vi "Dymin_FPGA_Main.vi"() -> ()   [LabVIEW 2016]
doc: "This VI demonstrates how to use an external signal to control the execution rate of a while loop."
uses:
  <vilib>/Platform/TimedLoop/XDataNode/timing_clust.ctl
  <vilib>/Platform/TimedLoop/XDataNode/nitl_modes.ctl
  <vilib>/Platform/TimedLoop/XDataNode/wakeup.ctl
  <vilib>/rvi/Emulation/niFpgaGetClockAttributes.vi
  <vilib>/rvi/Emulation/niFpgaSctlEmulationGetInTimedLoop.vi
  <vilib>/rvi/Emulation/niFpgaEmulationReportErrorSimple.vi
  <vilib>/rvi/eio/common/nirviEmuTemplateMethod_errors.vi
  <vilib>/rvi/Emulation/niFpgaCriticalErrorInLSC.vi
  <vilib>/rvi/Emulation/niFpgaEmulationIsFPGAContextNoSignature.vi
  <vilib>/rvi/errors/niFpgaSetErrorForExecOnDevCompSimple.vi
  <vilib>/rvi/eio/common/nirviEmuReportErrorAndStop.vi
  <vilib>/rvi/DataTransferAndStorage/Container/Common/niFpgaContainerGetUniqueNameForEmu.vi
  <vilib>/rvi/FIFO/Fifo_Resource/nirvififoEmulationSetSize.vi
  <vilib>/rvi/FIFO/Fifo_Resource/nirviFifoEmulationQueueMgr.vi
  <instcachedir>/0/nirviFifoEmulationQueueMgr_E5CAEC123FF24DC58D834DCA3CDAA9B5.lvgen/nirviFifoEmulationQueueMgr_E5CAEC123FF24DC58D834DCA3CDAA9B5_001.vi
  <vilib>/rvi/FIFO/Fifo_Resource/nirvififoEmulationDetermineInputValidOut.vi
  <vilib>/rvi/FIFO/Fifo_Resource/nirvififoEmulationCreateLock.vi
  <vilib>/rvi/Emulation/niFpgaProcessEmulError.vi
  <vilib>/rvi/FIFO/Fifo_Resource/nirvififoEmulationObtainLock.vi
  <vilib>/rvi/FIFO/Fifo_Resource/nirvififoEmulationReleaseLock.vi
  <vilib>/rvi/occurrence/nirviWaitOnOccurrenceBase.vi
  <vilib>/rvi/errors/nirviReportUnexpectedCaseInternalError.vi
  <vilib>/rvi/errors/nirviReportUnexpectedCaseInternalError (U32).vi
  <vilib>/Utility/error.llb/Clear Errors.vi
  <vilib>/rvi/interface/RandomDataEmulation/niFpgaRandomDataHandleErrors.vi
  <vilib>/eio/EIONode/EIONode.xnode
  <vilib>/Platform/TimedLoop/XDataNode/XDataNode.xnode
  <vilib>/rvi/DataTransferAndStorage/Container/XNode/niFpgaContainer.xnode
  <vilib>/rvi/FIFO/Fifo_Resource/nirvififoEmulationWrite.vi
  <vilib>/rvi/FIFO/Fifo_Resource/nirvififoEmulationRead.vi
  <vilib>/rvi/interface/RandomDataEmulation/nirviRandomDataFpgaReadWriteTemplate.vi
  <vilib>/Platform/TimedLoop/XDataNode/XDNodeRunTimeDep.lvlib
panel:
  in  "T3":u32=1000
  in  "T2":u32=1000
  in  "T1":u32=1000
  in  "T0":u32=1000
  in  "t3":u32=1000
  in  "t2":u32=1000
  in  "t1":u32=1000
  in  "t0":u32=1000
  in  "V3":u16=1000
  in  "V2":i16=1000
  in  "V1":i16=232
  in  "V0":u16=1000
  out "Overflow1":bool
  in  "Upper Threhold (counts)":u32
  out "Overflow2":bool
  out "PIX CLK (bits)":u32
  in  "Dymin On?":bool
  in  "stop 4":bool
  in  "stop 3":bool
  in  "stop 2":bool
  in  "stop 1":bool
  # "Reminder:These \"Volts\" are actually in bits.  Use  the RT_Main vi to run this code by inputting actual Volts.  Floats aren't possible in an FPGA program."
  # "Step before step with tn=0 is the last Dymin Step, threshold is ignored on last step, just count APD counts in selected time"
  # "AOM Voltage (bits)"
  # "Times (#80MHz periods)"
  # "Threshold (counts)"
  # "16=200ns\n32=400ns"
  # "nominal 12 bit ADC volts"
  # ".1=82\n.2=164\n.3=246"
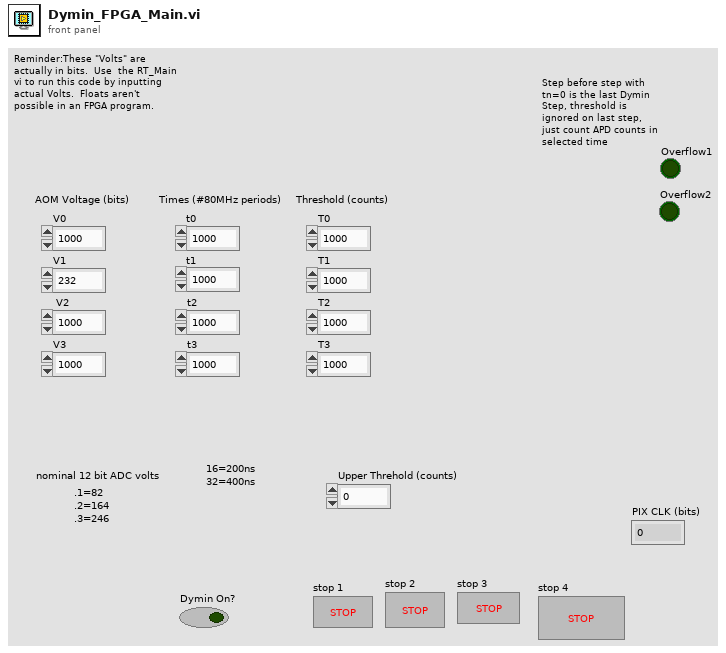
[diagram p1: front panel]
types:
  T1 = typedef "XDNodeRunTimeDep.lvlib/timing_clust.ctl" = cluster{"Expected End [f-1]":u64, "Actual End [f-1]":u64, "Finished Late? [f-1]":bool, "Expected End [i-1]":u64, "Actual End [i-1]":u64, "Finished Late? [i-1]":bool, "Expected Start [i]":u64, "Actual Start [i]":u64, "Expected Start [f]":u64, "Actual Start [f]":u64, "Source Name":string, "Structure Name":string, "Period":i64, "Deadline":i64, "Offset":i64, "Start":i64, "Priority":i32, "Timeout":i32, "Mode":T2, "Wakeup Reason":T3, "Error":errorcluster, "Source Type":string, "Secondary Source Type":string, "Global End Time":u64, "Global Start Time":u64, "Frame Duration":u64, "Iteration Duration":u64, "Assigned CPU":i32, "I/O Scan Engine Mode":u32}
  T2 = typedef "XDNodeRunTimeDep.lvlib/nitl_modes.ctl" = enum32{"No Change", "Process missed periods, maintain original phase", "Discard missed periods, maintain original phase", "Process missed periods, ignore original phase", "Discard missed periods, ignore original phase"}
  T3 = typedef "XDNodeRunTimeDep.lvlib/wakeup.ctl" = enum32{"Normal", "Aborted", "Asynchronous wakeup", "Timing source error", "Timed loop error", "Timeout"}
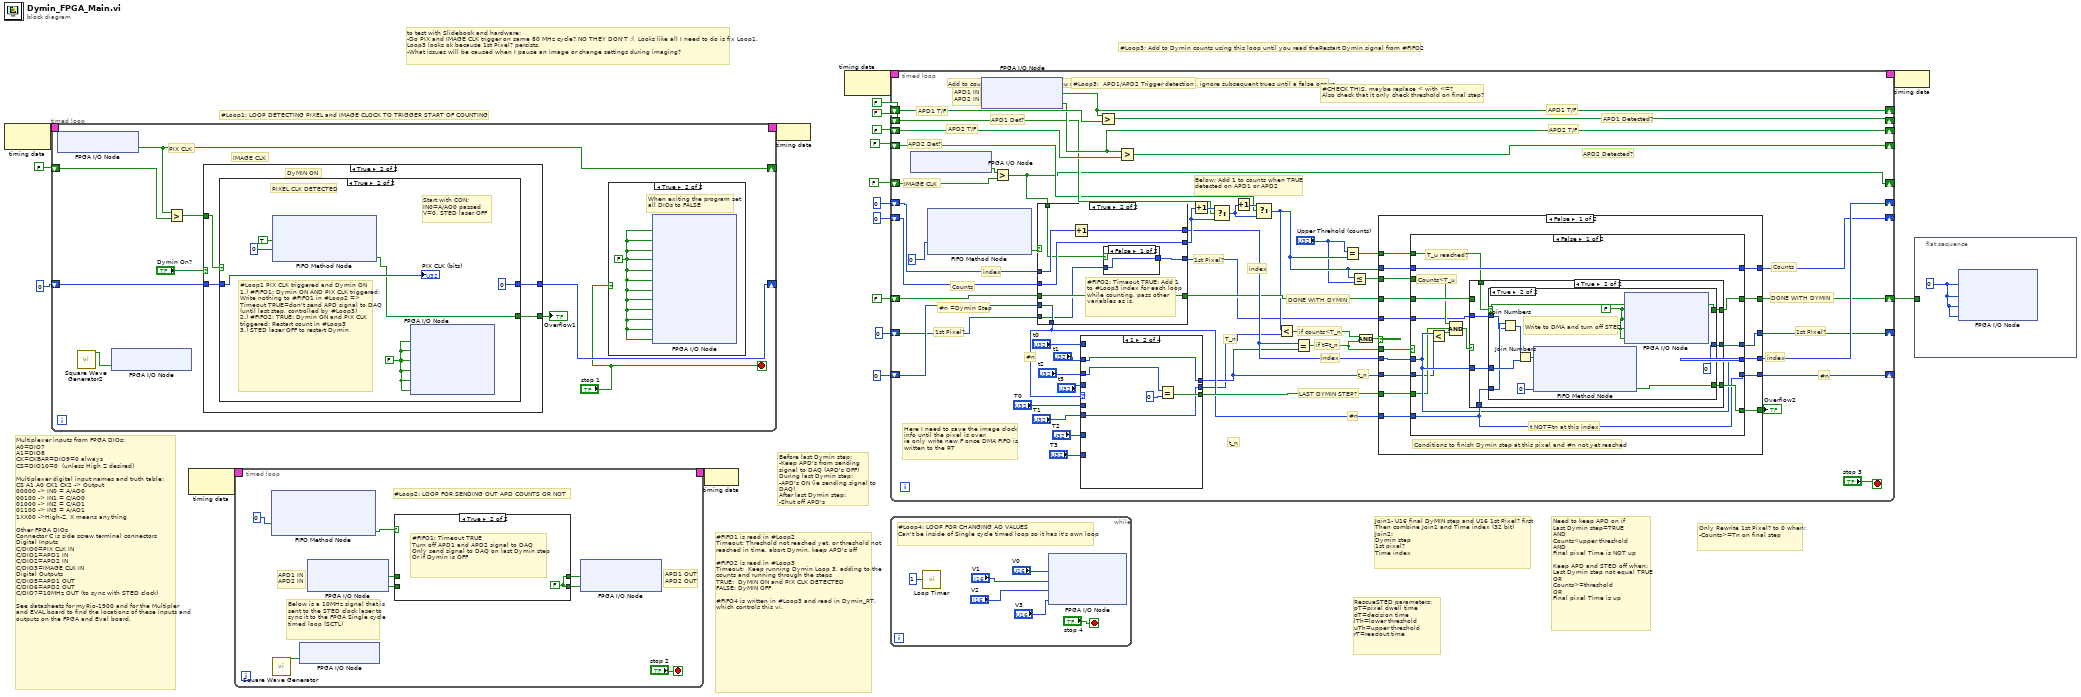
[diagram p0: block diagram]
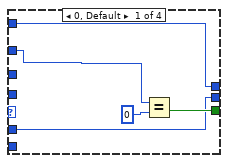
[diagram p2: hidden frame]
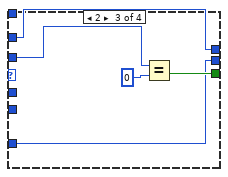
[diagram p3: hidden frame]
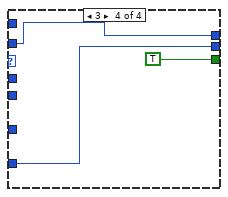
[diagram p4: hidden frame]
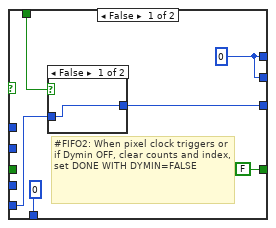
[diagram p5: hidden frame]
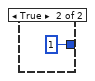
[diagram p6: hidden frame]
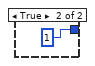
[diagram p7: hidden frame]
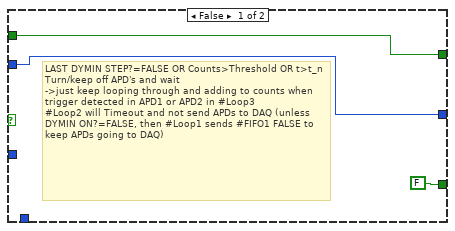
[diagram p8: hidden frame]
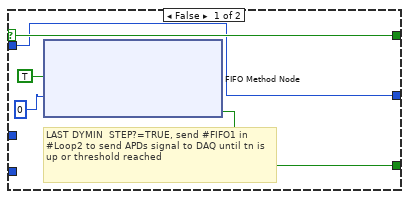
[diagram p9: hidden frame]
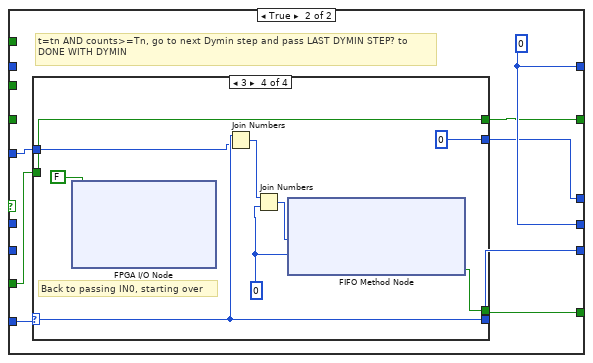
[diagram p10: hidden frame]
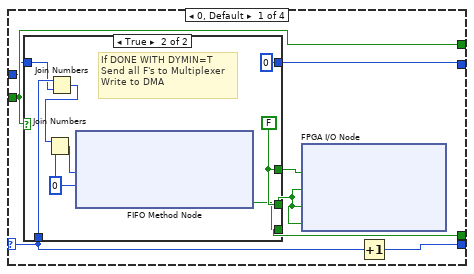
[diagram p11: hidden frame]
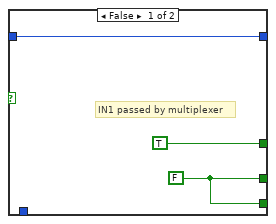
[diagram p12: hidden frame]
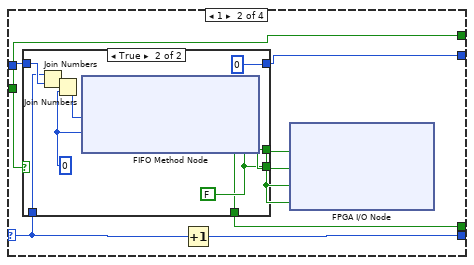
[diagram p13: hidden frame]
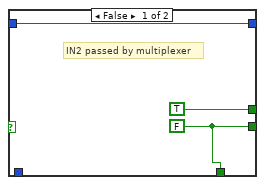
[diagram p14: hidden frame]
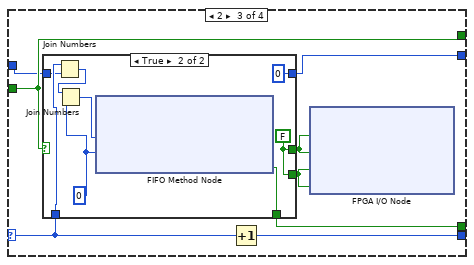
[diagram p15: hidden frame]
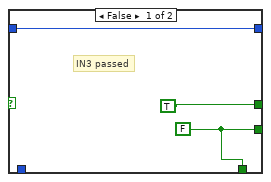
[diagram p16: hidden frame]
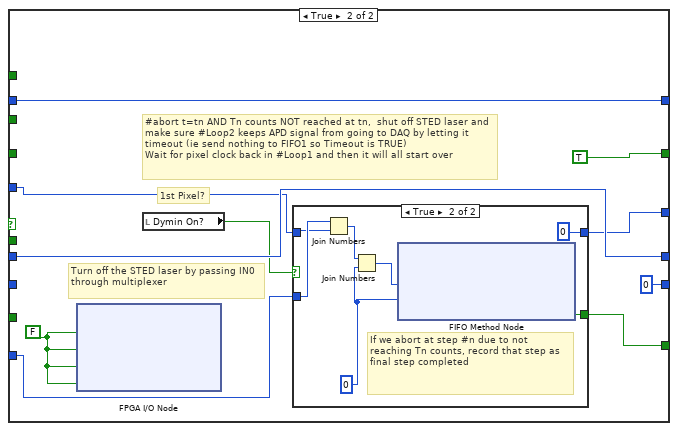
[diagram p17: hidden frame]
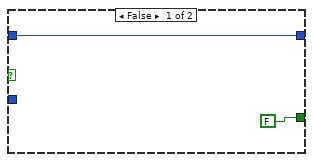
[diagram p18: hidden frame]
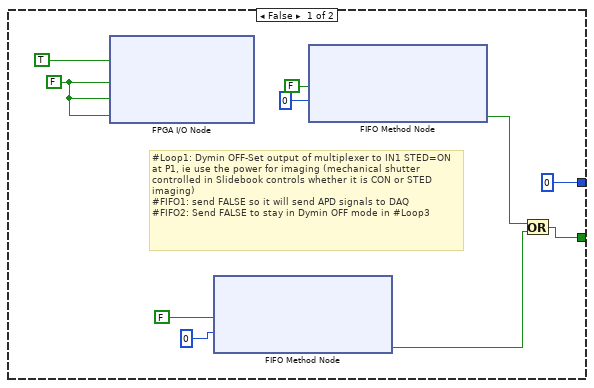
[diagram p20: hidden frame]
diagram:
  # "Only Rewrite 1st Pixel? to 0 when:\n-Counts>=Tn on final step"
  # "Join1- U16 final DyMIN step and U16 1st Pixel? first\nThen combine Join1 and Time index (32 bit)\nJoin2:\nDymin step\n1st pixel?\nTime index"
  # "Need to keep APD on if \nLast Dymin step=TRUE\nAND\nCounts<upper threshold\nAND\nFinal pixel Time is NOT up\n\nKeep APD and STED off when:\nLast Dymin step not equal TRUE\nOR\nCounts>=threshold\nOR\nFinal pixel Time is up"
  # "#Loop1: LOOP DETECTING PIXEL and IMAGE CLOCK TO TRIGGER START OF COUNTING"
  # "to test with Slidebook and hardware:\n-Do PIX and IMAGE CLK trigger on same 80 MHz cycle? NO THEY DON'T :(  Looks like all I need to do is fix Loop1, Loop3 looks ok because 1st Pixel? persists.\n-What issues will be caused when I pause an image or change settings during imaging?"
  # "Multiplexer inputs from FPGA DIOs:\nA0=DIO7\nA1=DIO8\nCK=CKBAR=DIO9=0 always\nCS=DIO10=0  (unless High Z desired)\n\nMultiplexer digital input names and truth table:\nCS A1 A0 CK1 CK2 -> Output\n00000 -> IN0 = A/AO0\n00100 -> IN1 = C/AO0\n01000 -> IN2 = C/AO1\n01100 -> IN3 = A/AO1\n1XX00 ->High-Z, X means anything\n\nOther FPGA DIOs\nConnector C is side screw terminal connectors\nDigital Inputs\nC/DIO0=PIX CLK IN\nC/DIO1=APD1 IN\nC/DIO2=APD2 IN\nC/DIO3=IMAGE CLK IN\nDigital Outputs\nC/DIO5=APD1 OUT\nC/DIO6=APD2 OUT\nC/DIO7=10MHz OUT (to sync with STED clock)\n\nSee datasheets for myRio-1900 and for the Multipler and EVAL board to find the locations of these inputs and outputs on the FPGA and Eval board."
  # "#FIFO1 is read in #Loop2\nTimeout: Threshold not reached yet, or threshold not reached in time, abort Dymin, keep APD's off\n\n#FIFO2 is read in #Loop3\nTimeout:  Keep running Dymin Loop 3, adding to the counts and running through the steps\nTRUE:  DyMIN ON and PIX CLK DETECTED\nFALSE: DyMIN OFF\n\n#FIFO4 is written in #Loop3 and read in Dymin_RT, which controls this vi."
  # "Before last Dymin step:\n-Keep APD's from sending signal to DAQ (APD's OFF)\nDuring last Dymin step:\n-APD's ON (ie sending signal to DAQ)\nAfter last Dymin step:\n-Shut off APD's"
  # "#Loop3: Add to Dymin counts using this loop until you read theRestart Dymin signal from #FIFO2"
  # "Add to counts using this loop until you read the FIRST TRUE value from the FIFO, ignore subsequent trues until a false occurs"
  # "RescueSTED parameters:\npT=pixel dwell time\ndT=decision time\nlTh=lower threshold\nuTh=upper threshold\nrT=readout time"
  n1 = node-c288() -> (w19:T1)  [unwired: 1 in]
  n2 = timed-loop {
    timing: w19 -> [_]
    timing-out: [_] -> w18
    shift-right: [w22] -> _
    shift-left: FALSE -> [w23]
    shift-right: [w26] -> _
    shift-left: u32 0 -> [w27]
    stop <- "stop 1" stop-if-true
    # "IMAGE CLK"
    # "PIX CLK"
    n3 = xnode "FPGA I/O Node"() -> ("ConnectorC/DIO0"=w22:bool)  [unwired: 1 in, 1 out]
    n4 = call "Square Wave Generator2"() -> ("square wave out"=w20:bool)  [unwired: 15 in]
    n5 = xnode "FPGA I/O Node"("ConnectorC/DIO4"=w20) -> ()  [unwired: 1 in, 1 out]
    n6 = Greater?(x=w22, y=w23) -> (0:w24:bool)
    n7 = case shown="True" "Dymin On?" {
      tunnel: w24 -> [_ w39]
      tunnel: w27 -> [_ w42]
      tunnel: [u32 0 w41] -> w26
      tunnel: [w30 w40] -> w25
      frame False {
        w37 = FALSE ("ConnectorA/DIO8")
        # "#Loop1: Dymin OFF-Set output of multiplexer to IN1 STED=ON at P1, ie use the power for imaging (mechanical shutter controlled in Slidebook controls whether it is CON or STED imaging)\n#FIFO1: send FALSE so it will send APD signals to DAQ \n#FIFO2: Send FALSE to stay in Dymin OFF mode in #Loop3"
        n8 = xnode "FPGA I/O Node"("ConnectorA/DIO7"=TRUE, "ConnectorA/DIO8"=w37, "ConnectorA/DIO9"=w37, "ConnectorA/DIO10"=w37) -> ()  [unwired: 4 in, 4 out]
        n9 = xnode ("FIFO Method Node")("Element"=FALSE, "Timeout"=0) -> ("Timed Out?"=w31:bool)  [unwired: 1 in, 1 out]
        n10 = xnode ("FIFO Method Node")("Element"=FALSE, "Timeout"=0) -> ("Timed Out?"=w32:bool)  [unwired: 1 in, 1 out]
        n11 = Or(x=w32, y=w31) -> (x .or. y?=w30:bool)
      }
      frame True {
        # "DyMIN ON"
        n12 = case shown="True" w39 {
          tunnel: w42 -> [w45 w49]
          tunnel: [w44 u32 0] -> w41
          tunnel: [FALSE ("Timed Out?") w48] -> w40
          frame False {
            # "#Loop1: No pixel clock trigger detected, don't do anything.  Loops 2 and 3 are working on Dymin for this pixel, just let them do their thing and you can just chill out loop 1.\nIf IMAGE CLK detected, pass 3 to #Loop3 with #FIFO2"
            n13 = Increment(x=w45) -> (x+1=w44:u32)
          }
          frame True {
            w51 = FALSE ("ConnectorA/DIO4")
            # "PIXEL CLK DETECTED"
            # "#Loop1 PIX CLK triggered and Dymin ON \n1.) #FIFO1: Dymin ON AND PIX CLK triggered: Write nothing to #FIFO1 in #Loop2 => Timeout TRUE=don't send APD signal to DAQ (until last step, controlled by #Loop3)\n2.) #FIFO2: TRUE: Dymin ON and PIX CLK triggered: Restart count in #Loop3\n3.) STED laser OFF to restart Dymin"
            # "Start with CON:\nIN0=A/AO0 passed\nV=0, STED laser OFF"
            n14 = xnode ("FIFO Method Node")("Element"=TRUE, "Timeout"=0) -> ("Timed Out?"=w48:bool)  [unwired: 1 in, 1 out]
            n15 = xnode "FPGA I/O Node"("ConnectorC/DIO5"=w51, "ConnectorC/DIO6"=w51, "ConnectorA/DIO7"=w51, "ConnectorA/DIO8"=w51, "ConnectorA/DIO9"=w51, "ConnectorA/DIO10"=w51) -> ()  [unwired: 6 in, 6 out]
            "PIX CLK (bits)" <- w49
          }
        }
      }
    }
    "Overflow1" <- w25
    n16 = case shown="True" "stop 1" {
      frame False {
      }
      frame True {
        w52 = FALSE
        # "When exiting the program set all DIOs to FALSE"
        n17 = xnode "FPGA I/O Node"("ConnectorC/DIO0"=w52, "ConnectorC/DIO1"=w52, "ConnectorC/DIO2"=w52, "ConnectorC/DIO3"=w52, "ConnectorC/DIO4"=w52, "ConnectorC/DIO5"=w52, "ConnectorC/DIO6"=w52, "ConnectorC/DIO7"=w52, "ConnectorA/DIO7"=w52, "ConnectorA/DIO8"=w52, "ConnectorA/DIO9"=w52, "ConnectorA/DIO10"=w52) -> ()  [unwired: 12 in, 12 out]
      }
    }
  }
  n18 = node-c288() -> (w16:T1)  [unwired: 1 in]
  n19 = timed-loop {
    timing: w16 -> [_]
    timing-out: [_] -> w15
    stop <- "stop 2" stop-if-true
    # "#Loop2: LOOP FOR SENDING OUT APD COUNTS OR NOT"
    # "Below is a 10MHz signal that is sent to the STED clock laser to sync it to the FPGA Single cycle timed loop (SCTL)"
    # "APD1 OUT\nAPD2 OUT"
    # "APD1 IN\nAPD2 IN"
    n20 = xnode ("FIFO Method Node")("Timeout"=0) -> ("Timed Out?"=w56:bool)  [unwired: 1 in, 2 out]
    n21 = call "Square Wave Generator"() -> ("square wave out"=w58:bool)  [unwired: 15 in]
    n22 = xnode "FPGA I/O Node"("ConnectorC/DIO7"=w58) -> ()  [unwired: 1 in, 1 out]
    n23 = xnode "FPGA I/O Node"() -> ("ConnectorC/DIO1"=w62:bool, "ConnectorC/DIO2"=w61:bool)  [unwired: 2 in, 2 out]
    n24 = case shown="True" w56 {
      tunnel: w62 -> [w64 _]
      tunnel: w61 -> [w63 _]
      tunnel: [w64 w65] -> w60
      tunnel: [w63 w65] -> w59
      frame False {
        # "#FIFO1: Timeout False (with element of TRUE OR FALSE): Last Dymin Step, send the signal to the DAQ for counting, or maybe just Dymin OFF=doing conventional CON or STED imaging, either way just pass it on."
      }
      frame True {
        w65 = FALSE
        # "#FIFO1: Timeout TRUE\nTurn off APD1 and APD2 signal to DAQ\nOnly send signal to DAQ on last Dymin step\nOr if Dymin is OFF"
      }
    }
    n25 = xnode "FPGA I/O Node"("ConnectorC/DIO5"=w60, "ConnectorC/DIO6"=w59) -> ()  [unwired: 2 in, 2 out]
  }
  n26 = node-c288(w15) -> ()
  n27 = node-c288(w18) -> ()
  n28 = node-c288() -> (w14:T1)  [unwired: 1 in]
  n29 = while {
    stop <- "stop 4" stop-if-true
    # "#Loop4: LOOP FOR CHANGING AO VALUES\nCan't be inside of Single cycle timed loop so it has it's own loop"
    n30 = call "Loop Timer"("Count(mSec)"=u32 1) -> ()  [unwired: 1 out]
    n31 = xnode "FPGA I/O Node"("ConnectorA/AO0"="V0", "ConnectorC/AO0"="V1", "ConnectorC/AO1"="V2", "ConnectorA/AO1"="V3") -> ()  [unwired: 4 in, 4 out]
  }
  n32 = timed-loop {
    timing: w14 -> [_]
    timing-out: [_] -> w13
    shift-right: [w122] -> _
    shift-left: FALSE -> [w124]
    shift-right: [w118] -> _
    shift-left: FALSE -> [w113]
    shift-right: [w108] -> _
    shift-left: u32 0 -> [w120]
    shift-right: [w106] -> _
    shift-left: FALSE -> [w114]
    shift-right: [w119] -> _
    shift-left: FALSE -> [w117]
    shift-right: [w107] -> _
    shift-left: u32 0 -> [w115]
    shift-right: [w110] -> _
    shift-left: u16 0 -> [w100]
    shift-right: [w103] -> w5
    shift-left: FALSE -> [w102]
    shift-right: [w87] -> _
    shift-left: u16 0 -> [w86]
    shift-right: [w74] -> _
    shift-left: FALSE -> [w75]
    stop <- "stop 3" stop-if-true
    # "IMAGE CLK"
    # "T_n"
    # "t_n"
    # "#CHECK THIS, maybe replace < with <=?\nAlso check that it only check threshold on final step?"
    # "1st Pixel?"
    # "1st PIxel?"
    # "1st Pixel?"
    # "Counts"
    # "index"
    # "Here I need to save the image clock\ninfo until the pixel is over,\nie only write new F once DMA FIFO is\nwritten to the RT"
    # "index"
    # "t_n"
    # "#n"
    # "#n"
    # "APD2 T/F"
    # "APD1 T/F"
    # "Below: Add 1 to counts when TRUE detected on APD1 or APD2"
    # "APD1 IN\nAPD2 IN"
    # "DONE WITH DYMIN"
    # "DONE WITH DYMIN"
    # "LAST DYMIN STEP?"
    # "#n =Dymin Step"
    # "#n"
    # "if counts<T_n"
    # "if t=t_n"
    # "index"
    # "APD1 Det?"
    # "APD2 Det?"
    # "APD2 Detected?"
    # "APD2 T/F"
    # "APD1 Detected?"
    # "APD1 T/F"
    # "index"
    # "Counts"
    # "#Loop3:  APD1/APD2 Trigger detection"
    n33 = xnode "FPGA I/O Node"() -> ("ConnectorC/DIO2"=w76:bool)  [unwired: 1 in, 1 out]
    n34 = xnode ("FIFO Method Node")("Timeout"=0) -> ("Timed Out?"=w95:bool)  [unwired: 1 in, 2 out]
    n35 = xnode "FPGA I/O Node"() -> ("ConnectorC/DIO1"=w122:bool, "ConnectorC/DIO2"=w119:bool)  [unwired: 2 in, 2 out]
    n36 = Greater?(x=w76, y=w75) -> (0:w74:bool)
    n37 = case shown="True" w95 {
      tunnel: [w143 w156] -> w121
      tunnel: [w143 w157] -> w109
      tunnel: w120 -> [_ w158]
      tunnel: w115 -> [_ w156]
      tunnel: w102 -> [_ w155]
      tunnel: [FALSE w155] -> w101
      tunnel: w100 -> [_ w154]
      tunnel: [u16 0 w154] -> w99
      tunnel: [w145 w151] -> w88
      tunnel: w86 -> [w144 w152]
      tunnel: w74 -> [w146 w153]
      frame False {
        w143 = u32 0
        # "#FIFO2: When pixel clock triggers or if Dymin OFF, clear counts and index, set DONE WITH DYMIN=FALSE"
        n38 = case shown="False" w146 {
          tunnel: [w149 u16 1] -> w145
          tunnel: w144 -> [w149 _]
          frame False {
          }
          frame True {
          }
        }
      }
      frame True {
        # "#FIFO2: Timeout TRUE: Add 1 to #Loop3 index for each loop while counting, pass other variables as is."
        n39 = Increment(x=w158) -> (x+1=w157:u32)
        n40 = case shown="False" w153 {
          tunnel: w152 -> [w159 _]
          tunnel: [w159 u16 1] -> w151
          frame False {
          }
          frame True {
          }
        }
      }
    }
    n41 = case shown="1" w99 {
      tunnel: [w127 w132 w137 w141] -> w89
      tunnel: [w128 w133 w138 TRUE] -> w105
      tunnel: [w125 w130 w135 w140] -> w85
      tunnel: "t0" -> [w127 _ _ _]
      tunnel: "t1" -> [w126 w132 _ _]
      tunnel: "t2" -> [_ w131 w137 _]
      tunnel: "t3" -> [_ _ w136 w141]
      tunnel: "T0" -> [w125 _ _ _]
      tunnel: "T1" -> [_ w130 _ _]
      tunnel: "T2" -> [_ _ w135 _]
      tunnel: "T3" -> [_ _ _ w140]
      frame 0, Default {
        n42 = Equal?(x=w126, y=u32 0) -> (x = y?=w128:bool)
      }
      frame 1 {
        n43 = Equal?(x=w131, y=u32 0) -> (x = y?=w133:bool)
      }
      frame 2 {
        n44 = Equal?(x=w136, y=u32 0) -> (x = y?=w138:bool)
      }
      frame 3 {
      }
    }
    n45 = Greater?(x=w122, y=w124) -> (0:w106:bool)
    n46 = Greater?(x=w119, y=w117) -> (0:w118:bool)
    n47 = Increment(x=w121) -> (x+1=w123:u32)
    n48 = Select(t=w123, s=w114, f=w121) -> (s? t:f=w97:u32)
    n49 = Increment(x=w97) -> (x+1=w116:u32)
    n50 = Select(t=w116, s=w113, f=w97) -> (s? t:f=w92:u32)
    n51 = Less?(x=w92, y=w85) -> (x < y?=w112:bool)
    n52 = Equal?(x=w109, y=w89) -> (x = y?=w104:bool)
    n53 = Equal?(x="Upper Threhold (counts)", y=w92) -> (x = y?=w93:bool)
    n54 = Less Or Equal?(x=w92, y="Upper Threhold (counts)") -> (x <= y?=w90:bool)
    n55 = And(x=w112, y=w104) -> (x .and. y?=w111:bool)
    n56 = case shown="False" w111 {
      tunnel: w99 -> [w176 w293]
      tunnel: [w165 u16 0] -> w110
      tunnel: w109 -> [w175 w298]
      tunnel: [w174 w298] -> w108
      tunnel: w92 -> [w172 w297]
      tunnel: [w173 w297] -> w107
      tunnel: w105 -> [w171 _]
      tunnel: w104 -> [w170 _]
      tunnel: [w169 TRUE] -> w103
      tunnel: w101 -> [w168 _]
      tunnel: [w167 w292] -> w96
      tunnel: w93 -> [w166 _]
      tunnel: w90 -> [w164 _]
      tunnel: w89 -> [w163 _]
      tunnel: w88 -> [w162 w291]
      tunnel: [w161 w290] -> w87
      frame False {
        # "Conditions to finish Dymin step at this pixel and #n not yet reached"
        n57 = case shown="False" w170 {
          tunnel: w176 -> [w186 w223]
          tunnel: w175 -> [w184 _]
          tunnel: [w184 w221] -> w174
          tunnel: [w190 w221] -> w173
          tunnel: w172 -> [w190 _]
          tunnel: w171 -> [w182 w222]
          tunnel: [w188 w220] -> w169
          tunnel: w168 -> [w185 _]
          tunnel: [w187 w219] -> w167
          tunnel: w166 -> [w189 _]
          tunnel: [w186 w218] -> w165
          tunnel: w164 -> [w181 _]
          tunnel: w163 -> [w179 _]
          tunnel: w162 -> [w178 w217]
          tunnel: [w177 w216] -> w161
          frame False {
            # "Counts<T_u"
            # "T_u reached?"
            # "t NOT=tn at this index"
            n58 = Less?(x=w184, y=w179) -> (x < y?=w183:bool)
            n59 = Compound Arithmetic op=AND(w181, w182, w183) -> (w180:bool)
            n60 = case shown="True" w180 {
              tunnel: w189 -> [_ w200]
              tunnel: w185 -> [w193 _]
              tunnel: [w193 w199] -> w188
              tunnel: [FALSE ("Timed Out?") w198] -> w187
              tunnel: w184 -> [_ w197]
              tunnel: w186 -> [_ w196]
              tunnel: w178 -> [w191 w195]
              tunnel: [w191 w194] -> w177
              frame False {
                # "LAST DYMIN STEP?=FALSE OR Counts>Threshold OR t>t_n\nTurn/keep off APD's and wait\n->just keep looping through and adding to counts when trigger detected in APD1 or APD2 in #Loop3\n#Loop2 will Timeout and not send APDs to DAQ (unless DYMIN ON?=FALSE, then #Loop1 sends #FIFO1 FALSE to keep APDs going to DAQ)"
              }
              frame True {
                n61 = case shown="True" w200 {
                  selector: w200 -> [w205 w215]
                  tunnel: [w205 w215] -> w199
                  tunnel: [w203 w211] -> w198
                  tunnel: w197 -> [_ w214]
                  tunnel: w196 -> [_ w210]
                  tunnel: w195 -> [w201 w209]
                  tunnel: [w201 u16 0] -> w194
                  frame False {
                    # "LAST DYMIN  STEP?=TRUE, send #FIFO1 in #Loop2 to send APDs signal to DAQ until tn is up or threshold reached"
                    n62 = xnode ("FIFO Method Node")("Element"=TRUE, "Timeout"=u8 0) -> ("Timed Out?"=w203:bool)  [unwired: 1 in, 1 out]
                  }
                  frame True {
                    w206 = FALSE ("ConnectorA/DIO7")
                    # "Write to DMA and turn off STED"
                    n63 = Join Numbers(hi=w210, lo=w209) -> ((hi.lo)=w208:u32)
                    n64 = Join Numbers(hi=w208, lo=w214) -> ((hi.lo)=w213:u64)
                    n65 = xnode "FIFO Method Node"("Element"=w213, "Timeout"=0) -> ("Timed Out?"=w211:bool)  [unwired: 1 in, 1 out]
                    n66 = xnode "FPGA I/O Node"("ConnectorA/DIO7"=w206, "ConnectorA/DIO8"=w206, "ConnectorA/DIO9"=w206, "ConnectorA/DIO10"=w206) -> ()  [unwired: 4 in, 4 out]
                  }
                }
              }
            }
          }
          frame True {
            w221 = u32 0
            # "t=tn AND counts>=Tn, go to next Dymin step and pass LAST DYMIN STEP? to DONE WITH DYMIN"
            n67 = case shown="3" w223 {
              selector: w223 -> [w227 w246 w265 w284]
              tunnel: [w231 w250 w269 w284] -> w218
              tunnel: w222 -> [w230 w249 w268 w288]
              tunnel: [w230 w249 w268 w288] -> w220
              tunnel: [w226 w245 w264 w287] -> w219
              tunnel: w217 -> [w225 w244 w263 w283]
              tunnel: [w224 w243 w262 u16 0] -> w216
              frame 0, Default {
                n68 = case shown="True" w230 {
                  tunnel: [TRUE ("ConnectorA/DIO7") w242] -> w229
                  tunnel: [w233 w242] -> w228
                  tunnel: w227 -> [_ w238]
                  tunnel: [w233 w241] -> w226
                  tunnel: w225 -> [w232 w237]
                  tunnel: [w232 u16 0] -> w224
                  frame False {
                    w233 = FALSE ("ConnectorA/DIO4")
                    # "IN1 passed by multiplexer"
                  }
                  frame True {
                    w240 = u32 0 ("Timeout")
                    w242 = FALSE
                    # "If DONE WITH DYMIN=T\nSend all F's to Multiplexer\nWrite to DMA"
                    n69 = Join Numbers(hi=w238, lo=w237) -> ((hi.lo)=w236:u32)
                    n70 = Join Numbers(hi=w236, lo=w240) -> ((hi.lo)=w239:u64)
                    n71 = xnode "FIFO Method Node"("Element"=w239, "Timeout"=w240) -> ("Timed Out?"=w241:bool)  [unwired: 1 in, 1 out]
                  }
                }
                n72 = xnode "FPGA I/O Node"("ConnectorA/DIO7"=w229, "ConnectorA/DIO8"=w228, "ConnectorA/DIO9"=w228, "ConnectorA/DIO10"=w228) -> ()  [unwired: 4 in, 4 out]
                n73 = Increment(x=w227) -> (x+1=w231:u16)
              }
              frame 1 {
                n74 = case shown="True" w249 {
                  tunnel: [w252 w261] -> w247
                  tunnel: [TRUE w261] -> w248
                  tunnel: w246 -> [_ w256]
                  tunnel: [w252 w260] -> w245
                  tunnel: w244 -> [w251 w257]
                  tunnel: [w251 u16 0] -> w243
                  frame False {
                    w252 = FALSE
                    # "IN2 passed by multiplexer"
                  }
                  frame True {
                    w259 = u32 0 ("Timeout")
                    w261 = FALSE
                    n75 = Join Numbers(hi=w256, lo=w257) -> ((hi.lo)=w254:u32)
                    n76 = Join Numbers(hi=w254, lo=w259) -> ((hi.lo)=w258:u64)
                    n77 = xnode "FIFO Method Node"("Element"=w258, "Timeout"=w259) -> ("Timed Out?"=w260:bool)  [unwired: 1 in, 1 out]
                  }
                }
                n78 = Increment(x=w246) -> (x+1=w250:u16)
                n79 = xnode "FPGA I/O Node"("ConnectorA/DIO7"=w247, "ConnectorA/DIO8"=w248, "ConnectorA/DIO9"=w247, "ConnectorA/DIO10"=w247) -> ()  [unwired: 4 in, 4 out]
              }
              frame 2 {
                n80 = case shown="True" w268 {
                  tunnel: [TRUE w280] -> w266
                  tunnel: [w271 w280] -> w267
                  tunnel: w265 -> [_ w276]
                  tunnel: [w271 w279] -> w264
                  tunnel: w263 -> [w270 w275]
                  tunnel: [w270 u16 0] -> w262
                  frame False {
                    w271 = FALSE
                    # "IN3 passed"
                  }
                  frame True {
                    w278 = u32 0 ("Timeout")
                    w280 = FALSE
                    n81 = Join Numbers(hi=w276, lo=w275) -> ((hi.lo)=w274:u32)
                    n82 = Join Numbers(hi=w274, lo=w278) -> ((hi.lo)=w277:u64)
                    n83 = xnode "FIFO Method Node"("Element"=w277, "Timeout"=w278) -> ("Timed Out?"=w279:bool)  [unwired: 1 in, 1 out]
                  }
                }
                n84 = Increment(x=w265) -> (x+1=w269:u16)
                n85 = xnode "FPGA I/O Node"("ConnectorA/DIO7"=w266, "ConnectorA/DIO8"=w266, "ConnectorA/DIO9"=w267, "ConnectorA/DIO10"=w267) -> ()  [unwired: 4 in, 4 out]
              }
              frame 3 {
                w285 = u32 0 ("Timeout")
                w289 = FALSE ("ConnectorA/DIO4")
                # "Back to passing IN0, starting over"
                n86 = xnode "FPGA I/O Node"("ConnectorA/DIO7"=w289, "ConnectorA/DIO8"=w289, "ConnectorA/DIO9"=w289, "ConnectorA/DIO10"=w289) -> ()  [unwired: 4 in, 4 out]
                n87 = Join Numbers(hi=w284, lo=w283) -> ((hi.lo)=w282:u32)
                n88 = Join Numbers(hi=w282, lo=w285) -> ((hi.lo)=w286:u64)
                n89 = xnode "FIFO Method Node"("Element"=w286, "Timeout"=w285) -> ("Timed Out?"=w287:bool)  [unwired: 1 in, 1 out]
              }
            }
          }
        }
      }
      frame True {
        w299 = FALSE
        # "1st Pixel?"
        # "Turn off the STED laser by passing IN0 through multiplexer"
        # "#abort t=tn AND Tn counts NOT reached at tn,  shut off STED laser and make sure #Loop2 keeps APD signal from going to DAQ by letting it timeout (ie send nothing to FIFO1 so Timeout is TRUE)\nWait for pixel clock back in #Loop1 and then it will all start over"
        n90 = xnode "FPGA I/O Node"("ConnectorA/DIO7"=w299, "ConnectorA/DIO8"=w299, "ConnectorA/DIO9"=w299, "ConnectorA/DIO10"=w299) -> ()  [unwired: 4 in, 4 out]
        n91 = local read "Dymin On?"() -> (w294:bool)
        n92 = case shown="True" w294 {
          tunnel: w293 -> [_ w305]
          tunnel: [FALSE ("Timed Out?") w308] -> w292
          tunnel: w291 -> [w300 w304]
          tunnel: [w300 u16 0] -> w290
          frame False {
          }
          frame True {
            w307 = u32 0
            # "If we abort at step #n due to not reaching Tn counts, record that step as final step completed"
            n93 = Join Numbers(hi=w305, lo=w304) -> ((hi.lo)=w303:u32)
            n94 = Join Numbers(hi=w303, lo=w307) -> ((hi.lo)=w306:u64)
            n95 = xnode "FIFO Method Node"("Element"=w306, "Timeout"=w307) -> ("Timed Out?"=w308:bool)  [unwired: 1 in, 1 out]
          }
        }
      }
    }
    "Overflow2" <- w96
  }
  n96 = node-c288(w13) -> ()
  n97 = flat-sequence {
    tunnel: w5 -> [_]
    frame #0 {
      w311 = u16 0 ("ConnectorA/AO0")
      n98 = xnode "FPGA I/O Node"("ConnectorA/AO0"=w311, "ConnectorA/AO1"=w311, "ConnectorC/AO0"=w311, "ConnectorC/AO1"=w311) -> ()  [unwired: 4 in, 4 out]
    }
  }
